vi "IconNumDotPoz(SubVI).vi"(9 "RangeChB":T1(ring) caption="Диапазон \"B\"", 10 "RangeChA":T2(ring) caption="Диапазон \"A\"", 11 "meas":string[](array[string])=["10:51:54", "244.889E-3", "175.506E-3", "23.235E+0", "15.882E+0", "10 В", "10 В"]) -> (3 "meas 2":string[](array[string])=["10:51:54", "244.889E-3", "175.506E-3", "23.235E+0", "15.882E+0", "10 В", "10 В"])   [LabVIEW 2017]
panel:
  out "resulting string":string
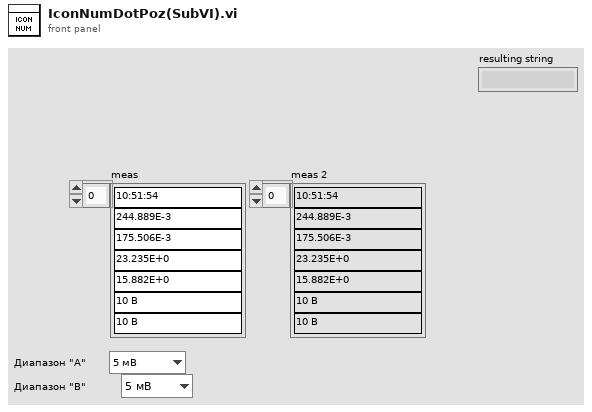
[diagram p1: front panel]
types:
  T1 = enum16{"5 мВ", "10 мВ", "25 мВ", "50 мВ", "100 мВ", "250 мВ", "0,5 В", "1 В", "2,5 В", "5 В", "10 В", "Авто", "Выкл."}
  T2 = enum16{"5 мВ", "10 мВ", "25 мВ", "50 мВ", "100 мВ", "250 мВ", "0,5 В", "1,0 В", "2,5 В", "5 В", "10 В", "Авто", "Выкл."}
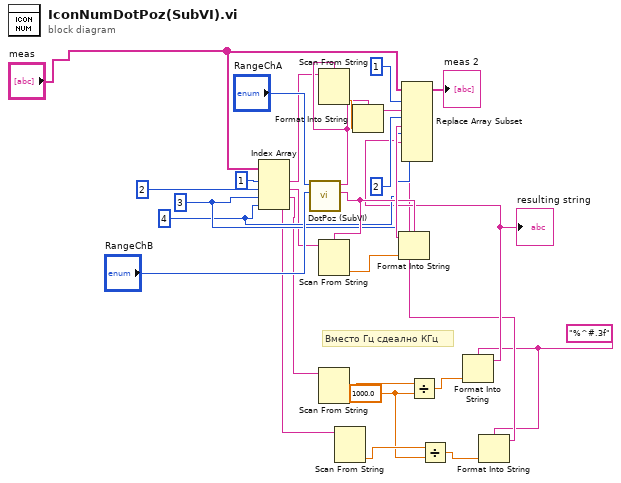
[diagram p0: block diagram]
diagram:
  w6 = "%^#.3f"
  w13 = 1000.0 ("y")
  w9 = 4 ("index")
  w10 = 3 ("index")
  # "Вместо Гц сдеално КГц"
  n1 = Index Array(array="meas", index #1=1 ("index"), index #2=2 ("index"), index #3=w10, index #4=w9) -> (element #1=w4:string, element #2=w3:string, element #3=w2:string, element #4=w1:string)
  n2 = call "DotPoz (SubVI).vi"("RangeChB"="RangeChB", "RangeChA"="RangeChA") -> ("Chanal B"=w16:string, "Chanal A"=w17:string)  [unwired: 6 in, 2 out]
  n3 = Scan From String(format string=w17, input string=w4) -> (output 1=w20:dbl)  [unwired: 3 in, 3 out]
  n4 = Scan From String(format string=w16, input string=w3) -> (output 1=w21:dbl)  [unwired: 3 in, 3 out]
  n5 = Scan From String(input string=w2) -> (output 1=w15:dbl)  [unwired: 4 in, 3 out]
  n6 = Scan From String(input string=w1) -> (output 1=w14:dbl)  [unwired: 4 in, 3 out]
  n7 = Format Into String(format string=w17, w20) -> (resulting string=w19:string)  [unwired: 2 in, 1 out]
  n8 = Format Into String(format string=w16, w21) -> (resulting string=w18:string)  [unwired: 2 in, 1 out]
  n9 = Divide(x=w15, y=w13) -> (x/y=w11:dbl)
  n10 = Divide(x=w14, y=w13) -> (x/y=w12:dbl)
  n11 = Format Into String(format string=w6, w11) -> (resulting string=w8:string)  [unwired: 2 in, 1 out]
  "resulting string" <- w8
  n12 = Format Into String(format string=w6, w12) -> (resulting string=w7:string)  [unwired: 2 in, 1 out]
  n13 = Replace Array Subset(array="meas", new element #1=w19, index #1=1 ("index"), new element #2=w18, index #2=2 ("index"), new element #3=w8, index #3=w10, new element #4=w7, index #4=w9) -> (→"meas 2":string[])
